vi "StatusMessages.vi"(1 "NewMessage":string, 2 "Status":string) -> (0 "AppendedMessage":string)   [LabVIEW 2010]
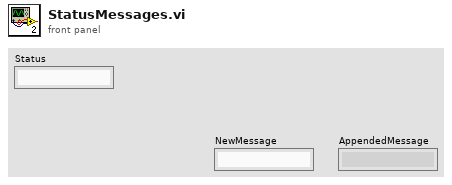
[diagram p1: front panel]
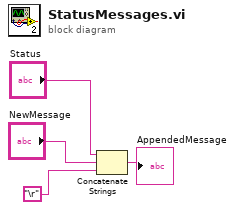
[diagram p0: block diagram]
diagram:
  n1 = Concatenate Strings("Status", "NewMessage", "\r") -> (→"AppendedMessage":string)
